vi "LiftMain.vi"(6 "Invert?":bool, 7 "Lift Power":dbl min=-1.0 max=1.0, 8 "error in (no error)":errorcluster, 9 "Reverse":bool, 10 "Forward":bool, 11 "Control Mode":enum16{"Open", "Control"}(ring)) -> (0 "error out":errorcluster, 2 "Output":dbl)   [LabVIEW 2016]
uses:
  <vilib>/Rock Robotics/SystemInterfaces/DIO/FPGA_DIOPWMChannel.ctl
  <vilib>/Rock Robotics/WPI/MotorControl/WPI_MotorControlOpen SPARK.vi
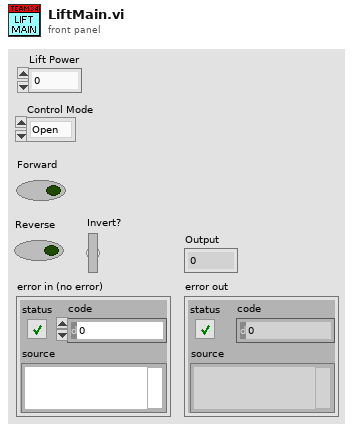
[diagram p1: front panel]
types:
  T1 = typedef "FPGA_DIOPWMChannel.ctl" = enum8{"PWM 0", "PWM 1", "PWM 2", "PWM 3", "PWM 4", "PWM 5", "PWM 6", "PWM 7", "PWM 8", "PWM 9", "PWM MXP 0", "PWM MXP 1", "PWM MXP 2", "PWM MXP 3", "PWM MXP 4", "PWM MXP 5", "PWM MXP 6", "PWM MXP 7", "PWM MXP 8", "PWM MXP 9", "Invalid"}
  T2 = typedef "WPI_MotorControlDeviceRef.ctl" = cluster{"DeviceStatus":errorcluster, "Type":T3, "PWM":cluster{"PWM Channel":T1, "DeadBand":T4}, "CAN":cluster{"Device Number":u8, "SetOutput VI Ref":variant, "GetOutput VI Ref":variant, "Enable VI Ref":variant, "Disable VI Ref":variant, "Data":variant}, "Invert":bool}
  T3 = typedef "WPI_MotorControlType.ctl" = enum16{"PWM", "CAN"}
  T4 = typedef "WPI_PWMDeadband.ctl" = cluster{"Name":string, "maxPositivePwm":i32, "minPositivePwm":i32, "centerPwm":i32, "maxNegativePwm":i32, "minNegativePwm":i32, "angularRange":u16}
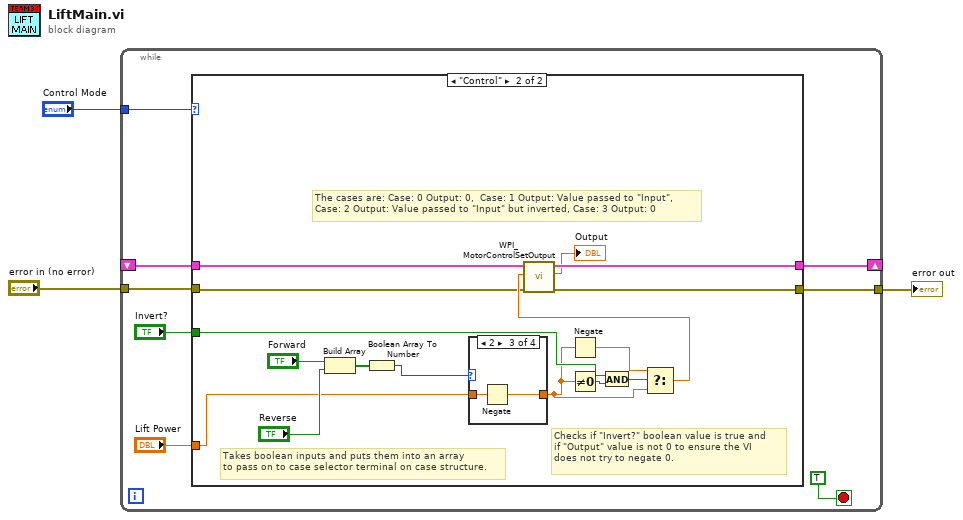
[diagram p0: block diagram]
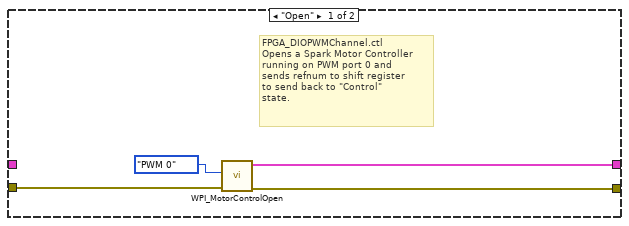
[diagram p2: hidden frame]
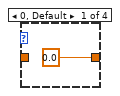
[diagram p3: hidden frame]
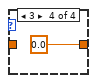
[diagram p5: hidden frame]
diagram:
  n1 = while {
    shift-right: [w9] -> _
    shift-left: _ -> [w8]
    tunnel: "Control Mode" -> [w10]
    tunnel: "error in (no error)" -> [w5]
    tunnel: [w4] -> w1
    stop <- TRUE stop-if-true
    n2 = case shown="\"Control\"" w10 {
      tunnel: [w15 w26] -> w9
      tunnel: w8 -> [_ w31]
      tunnel: "Lift Power" -> [_ w24]
      tunnel: "Invert?" -> [_ w22]
      tunnel: w5 -> [w13 w17]
      tunnel: [w12 w16] -> w4
      frame "Open" {
        # "FPGA_DIOPWMChannel.ctl\nOpens a Spark Motor Controller \nrunning on PWM port 0 and \nsends refnum to shift register \nto send back to \"Control\"\nstate."
        n3 = call-poly <vilib>:"WPI_MotorControlOpen.vi"("error in (no error)"=w13, "PWM Channel"=FPGA_DIOPWMChannel."PWM 0") -> ("error out"=w12:errorcluster, "MotorControlDeviceRef"=w15:T2)  [unwired: 8 in]
      }
      frame "Control" {
        # "Checks if \"Invert?\" boolean value is true and\nif \"Output\" value is not 0 to ensure the VI\ndoes not try to negate 0."
        # "Takes boolean inputs and puts them into an array\nto pass on to case selector terminal on case structure."
        # "The cases are: Case: 0 Output: 0,  Case: 1 Output: Value passed to \"Input\",\nCase: 2 Output: Value passed to \"Input\" but inverted, Case: 3 Output: 0"
        n4 = Build Array("Forward", "Reverse") -> (w28:bool[])
        n5 = Boolean Array To Number(Boolean array=w28) -> (number=w27:u32)
        n6 = case shown="2" w27 {
          tunnel: [0.0 w33 w34 0.0 ("Output")] -> w20
          tunnel: w24 -> [_ w33 w35 _]
          frame 0, Default {
          }
          frame 1 {
          }
          frame 2 {
            n7 = Negate(x=w35) -> (-x=w34:dbl)
          }
          frame 3 {
          }
        }
        n8 = Negate(x=w20) -> (-x=w25:dbl)
        n9 = Not Equal To 0?(x=w20) -> (x != 0?=w21:bool)
        n10 = And(x=w22, y=w21) -> (x .and. y?=w23:bool)
        n11 = Select(t=w25, s=w23, f=w20) -> (s? t:f=w18:dbl)
        n12 = call <vilib>:"WPI_MotorControlSetOutput.vi"("error in (no error)"=w17, "Output"=w18, "MotorControlDevRef"=w31) -> ("error out"=w16:errorcluster, "Motor Output"=→"Output":dbl, "MotorControlDevRef"=w26:T2)  [unwired: 6 in]
      }
    }
  }
  "error out" <- w1
